vi "DataToEnv.vi"(2 "Name":string, 3 "Data":string[][](table), 4 "Env In":variant) -> (0 "Data Variant":variant, 1 "Env Out":variant)   [LabVIEW 2014]
uses:
  Env.global.vi
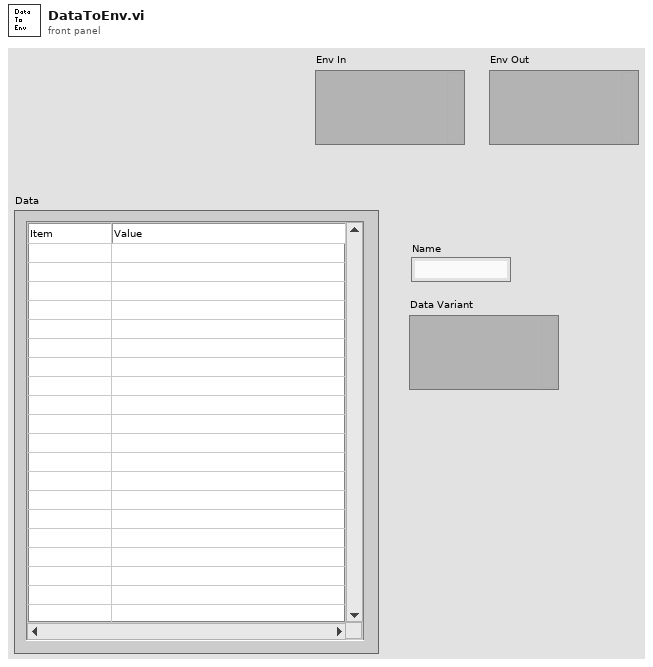
[diagram p1: front panel]
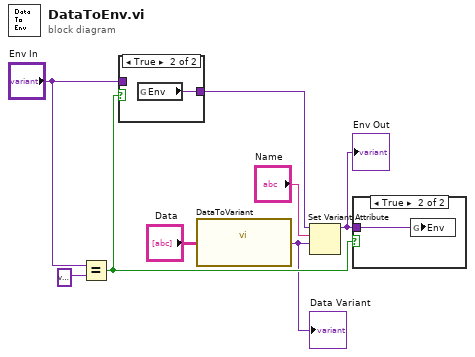
[diagram p0: block diagram]
diagram:
  n1 = Equal?(x="Env In", y=variant ("Env In")) -> (x = y?=w4:bool)
  n2 = case shown="True" w4 {
    tunnel: [w9 w10] -> w6
    tunnel: "Env In" -> [w9 _]
    frame False {
    }
    frame True {
      n3 = global read "Env.global.vi" "Env"() -> (w10:variant)
    }
  }
  n4 = call "DataToVariant.vi"("Data"="Data") -> ("Variant"=w1:variant)
  "Data Variant" <- w1
  n5 = Set Variant Attribute(Variant=w6, name="Name", value=w1) -> (Variant out=w3:variant)  [unwired: 1 in, 2 out]
  "Env Out" <- w3
  n6 = case shown="True" w4 {
    tunnel: w3 -> [_ w11]
    frame False {
    }
    frame True {
      n7 = global write "Env.global.vi" "Env"(w11) -> ()
    }
  }
